vi "Letter Mouse Down.vi"(11 "Letter_Ref":refnum<vi>) -> ()   [LabVIEW 2015]
uses:
  TypeDef/Color.ctl
panel:
  in  "Color":T1=12369084 items=["Free"=9567230, "Letter"=16774186, "Any"=16448250, "Exclude"=12369084]
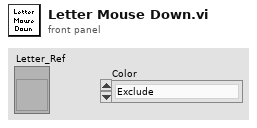
[diagram p1: front panel]
types:
  T1 = typedef "Color.ctl" = u32
  T2 = typedef "LVStringsAndValuesArrayTypeDef_U32.ctl" = cluster{"String":string, "Value":u32}[]
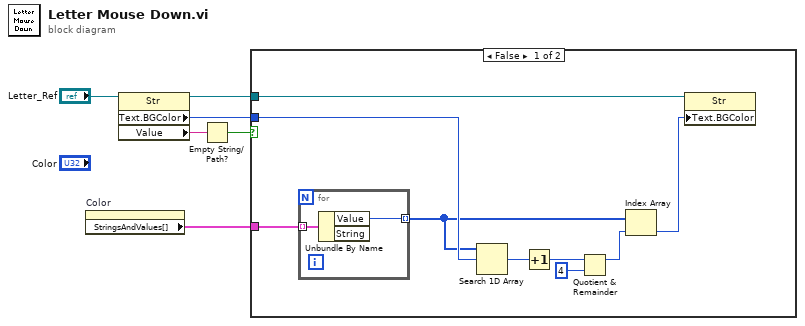
[diagram p0: block diagram]
diagram:
  n1 = property on="Color" class="Ring (strict)"() -> ("StringsAndValues[]"=w4:T2)  [unwired: 2 in, 2 out]
  n2 = property class="Str"(reference="Letter_Ref") -> (reference out=w6:refnum<vi>, "Text.BGColor"=w3:u32, "Value"=w2:string)  [unwired: 1 in, 1 out]
  n3 = Empty String/Path?(string/path=w2) -> (empty?=w1:bool)
  n4 = case shown="False" w1 {
    tunnel: w6 -> [w15 _]
    tunnel: w4 -> [w14 _]
    tunnel: w3 -> [w13 _]
    frame False {
      n5 = for {
        tunnel: w14 -> [w17] mode=indexing
        tunnel: [w16] -> w9 mode=indexing
        n6 = Unbundle By Name(w17) -> ("Value"=w16:u32)  [unwired: 1 out]
      }
      n7 = Search 1D Array(1D array=w9, element=w13) -> (index of element=w12:i32)  [unwired: 1 in]
      n8 = Increment(x=w12) -> (x+1=w11:i32)
      n9 = Quotient & Remainder(x=w11, y=4) -> (x-y*floor(x/y)=w8:i32)  [unwired: 1 out]
      n10 = Index Array(array=w9, index=w8) -> (element=w7:u32)
      n11 = property class="Str"(reference=w15, "Text.BGColor"=w7) -> ()  [unwired: 1 in, 2 out]
    }
    frame True {
    }
  }
